vi "remote.Read Dev.ProductName.vi"(8 "error in (no error)":errorcluster, 11 "SLSC Remote in":refnum<class "SLSC Interface.lvclass">) -> (0 "error out":errorcluster, 2 "Dev.ProductName":string, 3 "SLSC Remote out":refnum<class "SLSC Interface.lvclass">)   [LabVIEW 2016, in "SLSC Interfaces.lvlib" / "SLSC Interface.lvclass"]
uses:
  SLSC Interface Class/SLSC Interface.lvclass
  <vilib>/NI/JSON Support for LabVIEW/JSON Data Classes/JSON Helper/To More Specific Type (String).vi
  <vilib>/NI/JSON Support for LabVIEW/JSON Data Classes/JSON String/Read value (String).vi
  <vilib>/NI/JSON Support for LabVIEW/JSON Data Classes/JSON Helper/JSON Helper.lvclass
  <vilib>/NI/JSON Support for LabVIEW/JSON Data Classes/JSON String/JSON String.lvclass
  <vilib>/NI/JSON Support for LabVIEW/JSON Data Classes/JSON Basic Type/JSON Literal.lvclass
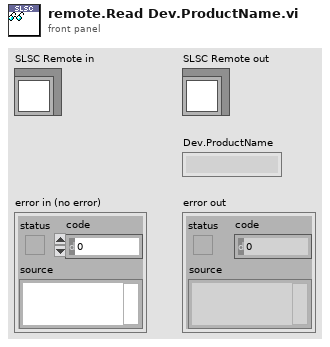
[diagram p1: front panel]
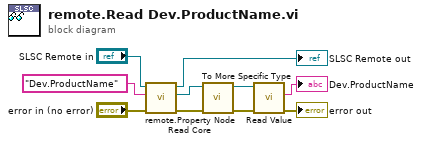
[diagram p0: block diagram]
diagram:
  n1 = call "remote.Property Node Read Core.vi"("error in (no error)"="error in (no error)", "property"="Dev.ProductName", "SLSC Remote in"="SLSC Remote in") -> ("error out"=w10:errorcluster, "value"=w5:refnum<class "JSON Null.lvclass">, "SLSC Remote out"=→"SLSC Remote out":refnum<class "SLSC Interface.lvclass">)  [unwired: 6 in]
  n2 = call-poly <vilib>:"To More Specific Type.vi"("error in (no error)"=w10, "JSON Datatype in"=w5) -> ("error out"=w6:errorcluster, "JSON Datatype out"=w2:refnum<class "JSON String.lvclass">)  [unwired: 8 in]
  n3 = call-poly <vilib>:"Read Value.vi"("error in (no error)"=w6, "JSON String in"=w2) -> ("error out"=→"error out":errorcluster, "value"=→"Dev.ProductName":string)  [unwired: 8 in]
